vi "TIFF-Append Tag (U32).vi"(0 "IFD in":u8[](array[numeric]), 5 "[IN] TagID":u16, 7 "[IN] DataType":u16(ring)=4 items=["BYTE"=1, "ASCII"=2, "SHORT"=3, "LONG"=4, "RATIONAL"=5], 9 "[IN] Data":u32, 11 "error IN":errorcluster, 12 "[IN] Byte order":T1(ring)) -> (4 "IFD out":u8[](array[numeric]), 15 "error OUT":errorcluster)   [LabVIEW 2020]
doc: "This VI writes a tif TAG. Input data is an array of U32. Note that the data should not be larger than 4 bytes."
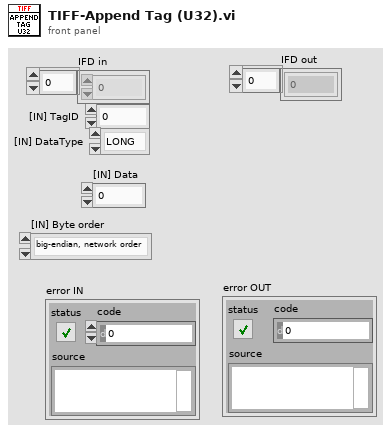
[diagram p1: front panel]
types:
  T1 = enum16{"big-endian, network order", "native, host order", "little-endian"}
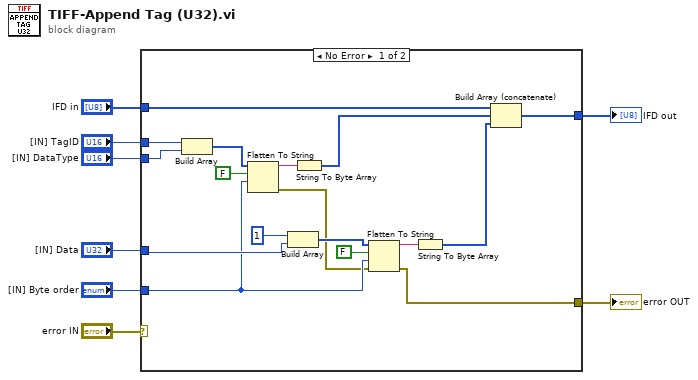
[diagram p0: block diagram]
diagram:
  n1 = case shown="No Error" "error IN" {
    selector: "error IN" -> [_ w27]
    tunnel: [w9 w27] -> w8
    tunnel: "[IN] Byte order" -> [w16 _]
    tunnel: "[IN] Data" -> [w20 _]
    tunnel: "[IN] TagID" -> [w25 _]
    tunnel: "[IN] DataType" -> [w24 _]
    tunnel: "IFD in" -> [w14 w26]
    tunnel: [w11 w26] -> w1
    frame No Error {
      n2 = Build Array(w25, w24) -> (w21:u16[])
      n3 = Flatten To String(anything=w21, prepend array or string size? (T)=FALSE, byte order (0:big-endian, network order)=w16) -> (data string=w23:string, error out=w10:errorcluster)  [unwired: 1 in, 1 out]
      n4 = Build Array(u32 1 ("[IN] Data"), w20) -> (w15:u32[])
      n5 = String To Byte Array(string=w23) -> (unsigned byte array=w13:u8[])
      n6 = Flatten To String(anything=w15, prepend array or string size? (T)=FALSE, byte order (0:big-endian, network order)=w16, error in (no error)=w10) -> (data string=w18:string, error out=w9:errorcluster)  [unwired: 1 out]
      n7 = String To Byte Array(string=w18) -> (unsigned byte array=w12:u8[])
      n8 = Build Array (concatenate)(w14, w13, w12) -> (w11:u8[])
    }
    frame Error {
    }
  }
  "error OUT" <- w8
  "IFD out" <- w1
